vi "样品下电.vi"(6 "error in (no error)":errorcluster, 9 "仪器实例 out":T1) -> (0 "error out":errorcluster, 3 "仪器实例 out 2":T1)   [LabVIEW 2020]
uses:
  F:/F020/S7_1200 control/HslCommunication.dll
  S7_1200 control/HslCommunication.dll
  S7_1200 control/S7_1200 WriteBools.vi
  <instrlib>/TDK-Lambda G Series/TDK-Lambda G Series.lvlib
  <instrlib>/IT6300/IT6300.lvlib
  S7_1200 control/S7_1200 control.lvlib
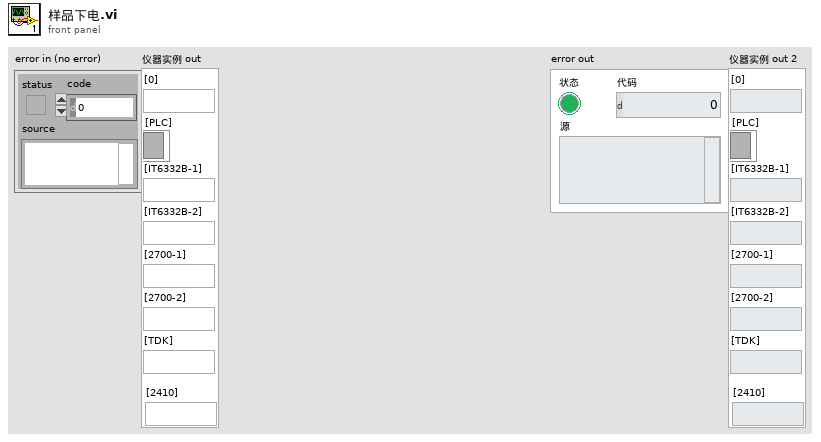
[diagram p1: front panel]
types:
  T1 = typedef "仪器实例.ctl" = cluster{"[0]":string, "[PLC]":refnum<k24>, "[IT6332B-1]":string, "[IT6332B-2]":string, "[2700-1]":string, "[2700-2]":string, "[TDK]":string, "[2410]":string}
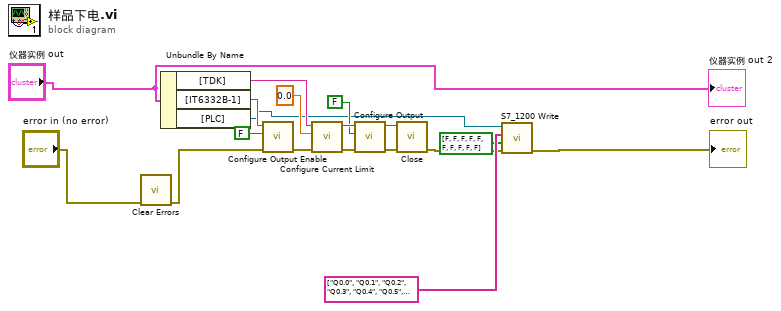
[diagram p0: block diagram]
diagram:
  n1 = call <vilib>:"Clear Errors.vi"("error in (no error)"="error in (no error)") -> ("error out"=w1:errorcluster)  [unwired: 5 in, 1 out]
  n2 = Unbundle By Name("仪器实例 out") -> ("[TDK]"=w9:string, "[IT6332B-1]"=w11:string, "[PLC]"=w4:refnum<k24>)
  n3 = call <instrlib>:"Configure Output Enable.vi"("error in (no error)"=w1, "Enable Output (T: Enable)"=FALSE, "VISA resource name"=w11) -> ("error out"=w8:errorcluster)  [unwired: 7 in, 1 out]
  n4 = call <instrlib>:"Configure Current Limit.vi"("error in (no error)"=w8, "Current Limit (0A)"=0.0, "VISA resource name"=w9) -> ("error out"=w13:errorcluster, "VISA resource name out"=w14:refnum<visa-resource-name>)  [unwired: 7 in]
  n5 = call <instrlib>:"Configure Output.vi"("error in (no error)"=w13, "Enable Output (False)"=FALSE, "VISA resource name"=w14) -> ("error out"=w7:errorcluster, "VISA resource name out"=w6:refnum<visa-resource-name>)  [unwired: 7 in]
  n6 = call <instrlib>:"Close.vi"("error in (no error)"=w7, "VISA resource name"=w6) -> ("error out"=w5:errorcluster)  [unwired: 9 in]
  n7 = call-poly "S7_1200 Write.vi"("错误输入（无错误）"=w5, "values"=bool[] [FALSE, FALSE, FALSE, FALSE, FALSE, FALSE, FALSE, FALSE, FALSE, FALSE], "addresses"=string[] ["Q0.0", "Q0.1", "Q0.2", "Q0.3", "Q0.4", "Q0.5", "Q0.6", "Q0.7", "Q1.0", "Q1.1"], "引用"=w4) -> ("错误输出"=→"error out":errorcluster)  [unwired: 2 in, 1 out]
  "仪器实例 out 2" <- "仪器实例 out"
